vi "Inspect Init Global Variable Values.vi"(11 "Inspection Name":string) -> ()   [LabVIEW 2019]
uses:
  Common.llb/IVB Variable Data Cluster.ctl
  <vilib>/vision/Image Controls.llb/IMAQ Image.ctl
  Common.llb/IVB Global Variable - Manager Mode.ctl
  kernel32.dll
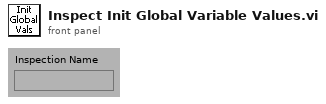
[diagram p1: front panel]
types:
  T1 = typedef "IVB Global Variable - Manager Mode.ctl" = enum16{"Init", "Delete User Defined", "Update User Defined", "Get All User Defined", "Get All System", "Set Current Value System", "Set Current Value User Defined", "Add/Update Variable"}
  T2 = typedef "IVB Variable Data Cluster.ctl" = cluster{"String":string, "Numeric":dbl, "Boolean":bool, "Point":cluster{"X":dbl, "Y":dbl}, "Image":T3, "1D String":string[], "1D Numeric":dbl[], "1D Boolean":bool[]}
  T3 = typedef "IMAQ Image.ctl" = refnum<image>
  T4 = enum16{"Reset", "Start Process", "Suspend Process", "Add Elapsed Time", "Get Results"}
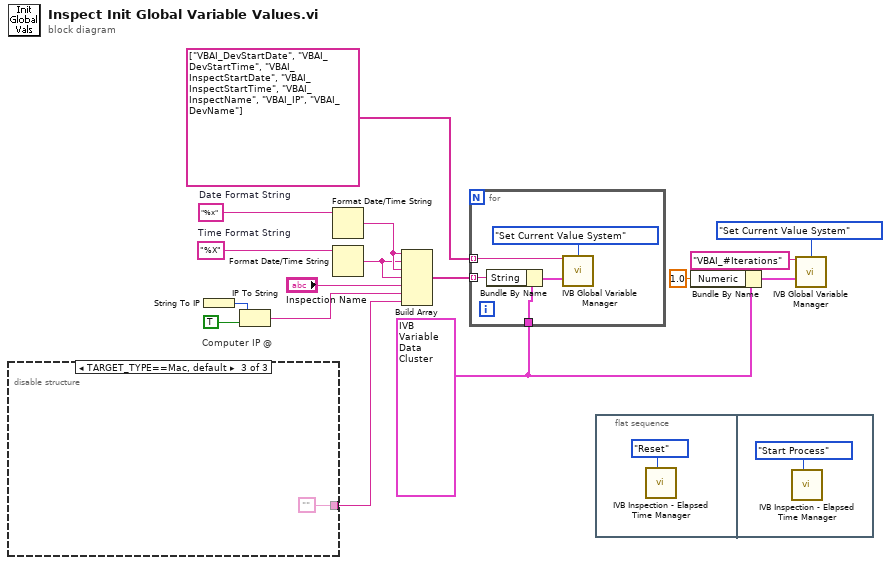
[diagram p0: block diagram]
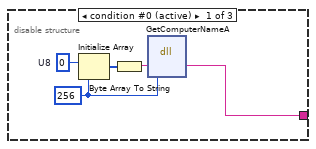
[diagram p2: hidden frame]
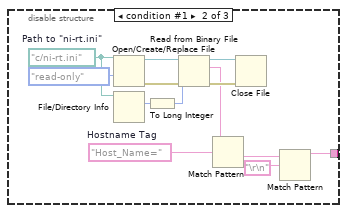
[diagram p3: hidden frame]
diagram:
  w2 = T2 {"String"="", "Numeric"=0.0, "Boolean"=FALSE, "Point"={"X"=0.0, "Y"=0.0}, "Image"=refnum, "1D String"=[], "1D Numeric"=[], "1D Boolean"=[]} ("Data In")
  w7 = "%X"  # Time Format String
  w6 = "%x"  # Date Format String
  # "Computer IP @"
  n1 = disable-structure shown="TARGET_TYPE==Mac, default" {
    disable-tunnel: [w17 w34 ""] -> w8
    frame condition #0 (active) {
      w19 = 256
      w18 = u8 0  # U8
      n2 = Initialize Array(w18, w19) -> (w21:u8[])
      n3 = Byte Array To String(unsigned byte array=w21) -> (string=w20:string)
      n4 = dll-call lib="kernel32.dll" fn="GetComputerNameA"(w20, w19) -> (w17:string)  [unwired: 5 in, 2 out]
    }
    frame condition #1 {
      w28 = "Host_Name="  # Hostname Tag
      w26 = path "c:/ni-rt.ini"  # Path to "ni-rt.ini"
      n5 = Open/Create/Replace File(file path (use dialog)=w26, access (0:read/write)=enum16{"read/write", "read-only", "write-only"}."read-only") -> (refnum out=w27:refnum<file>, error out=w32:errorcluster)  [unwired: 4 in, 1 out]
      n6 = File/Directory Info(path=w26) -> (size=w22:i64)  [unwired: 1 in, 6 out]
      n7 = To Long Integer(number=w22) -> (32bit integer=w25:i32)
      n8 = Read from Binary File(8:w32, 10:w25, 11:w27) -> (0:w30:errorcluster, 2:w29:string, 3:w31:refnum<file>)  [unwired: 3 in, 1 out]
      n9 = Match Pattern(string=w29, regular expression=w28) -> (after substring=w24:string)  [unwired: 1 in, 3 out]
      n10 = Close File(refnum=w31, error in=w30) -> ()  [unwired: 2 out]
      n11 = Match Pattern(string=w24, regular expression="\r\n") -> (before substring=w34:string)  [unwired: 1 in, 3 out]
    }
    frame condition #2 {
    }
  }
  n12 = String To IP() -> (0:w15:u32)  [unwired: 1 in]
  n13 = IP To String(1:TRUE ("dot notation? (F)"), 2:w15) -> (0:w11:string)
  n14 = Format Date/Time String(time format string (%c)=w6) -> (date/time string=w14:string)  [unwired: 2 in]
  n15 = Format Date/Time String(time format string (%c)=w7) -> (date/time string=w13:string)  [unwired: 2 in]
  n16 = Build Array(w14, w13, w14, w13, "Inspection Name", w11, w8) -> (w10:string[])
  n17 = for {
    tunnel: w10 -> [w37] mode=indexing
    tunnel: string[] ["VBAI_DevStartDate", "VBAI_DevStartTime", "VBAI_InspectStartDate", "VBAI_InspectStartTime", "VBAI_InspectName", "VBAI_IP", "VBAI_DevName"] -> [w39] mode=indexing
    tunnel: w2 -> [w38]
    n18 = Bundle By Name(cluster=w38, "String"=w37) -> (w36:T2)
    n19 = call "IVB Global Variable Manager.vi"("GUID"=w39, "Function"=IVB_Global_Variable_-_Manager_Mode."Set Current Value System", "Data In"=w36) -> ()  [unwired: 11 in, 2 out]
  }
  n20 = flat-sequence {
    frame #0 {
      n21 = call "IVB Inspection - Elapsed Time Manager.vi"("Function"=T4."Reset") -> ()  [unwired: 7 in, 4 out]
    }
    frame #1 {
      n22 = call "IVB Inspection - Elapsed Time Manager.vi"("Function"=T4."Start Process") -> ()  [unwired: 7 in, 4 out]
    }
  }
  n23 = Bundle By Name(cluster=w2, "Numeric"=1.0) -> (w3:T2)
  n24 = call "IVB Global Variable Manager.vi"("GUID"="VBAI_#Iterations", "Function"=IVB_Global_Variable_-_Manager_Mode."Set Current Value System", "Data In"=w3) -> ()  [unwired: 11 in, 2 out]
